vi "Configuration Voltage.vi"(0 "VISA resource name":refnum<visa-resource-name>, 5 "Channel 1-8 (0:Ch1)":u8(ring) items=["Channel 1", "Channel 2", "Channel 3", "Channel 4", "Channel 5", "Channel 6", "Channel 7", "Channel 8 "], 7 "Voltage Level (40.0V)":sgl=40.0 min=0 format="%.4f", 11 "error in (no error)":errorcluster, 12 "Response Speed (0:Slow)":u8(slide) scale=0.0..1.0, 13 "Current Limit (2.0A)":sgl=2.0 min=0 format="%.2f") -> (4 "VISA resource name out":refnum<visa-resource-name>, 15 "error out":errorcluster)   [LabVIEW 2015, in "Chroma ATE 6310.lvlib"]
doc: "This function sets the constant voltage mode.\n\nIn CV mode ,the Load will sink current to control the voltage source in programmed value."
uses:
  <instrlib>/Chroma ATE 6310/Chroma ATE 6310.lvlib
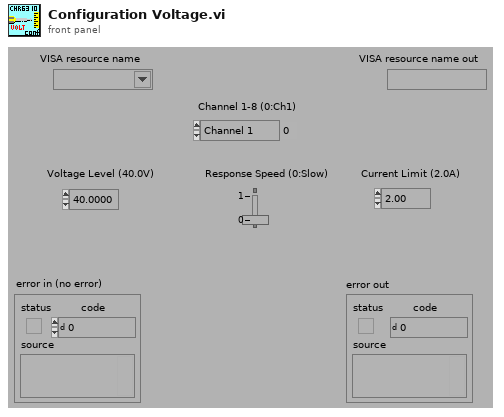
[diagram p1: front panel]
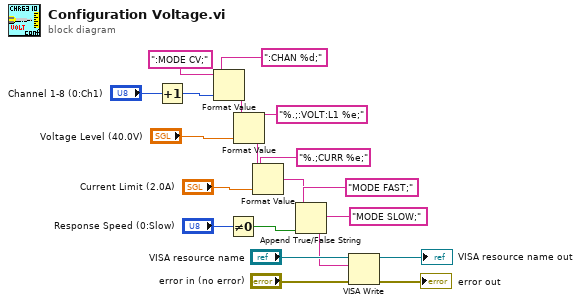
[diagram p0: block diagram]
diagram:
  n1 = Increment(x="Channel 1-8 (0:Ch1)") -> (x+1=w15:u8)
  n2 = Format Value(string ("")=":MODE CV;", format string=":CHAN %d;", value (0)=w15) -> (output string=w13:string)
  n3 = Not Equal To 0?(x="Response Speed (0:Slow)") -> (x != 0?=w19:bool)
  n4 = Format Value(string ("")=w13, format string="%.;:VOLT:L1 %e;", value (0)="Voltage Level (40.0V)") -> (output string=w10:string)
  n5 = Format Value(string ("")=w10, format string="%.;CURR %e;", value (0)="Current Limit (2.0A)") -> (output string=w11:string)
  n6 = Append True/False String(1:w19, 2:"MODE SLOW;", 3:"MODE FAST;", 4:w11) -> (0:w2:string)
  n7 = VISA Write(VISA resource name="VISA resource name", write buffer=w2, error in (no error)="error in (no error)") -> (VISA resource name out=→"VISA resource name out":refnum<visa-resource-name>, error out=→"error out":errorcluster)  [unwired: 1 out]
